vi "FL_Adjust_raw_magnets_coords.vi"(4 "Offset H.":sgl, 5 "Offset V.":sgl, 6 "Alternative magnets orientation":bool, 7 "DEC cluster in":T1) -> (1 "DEC cluster out":T1)   [LabVIEW 2018]
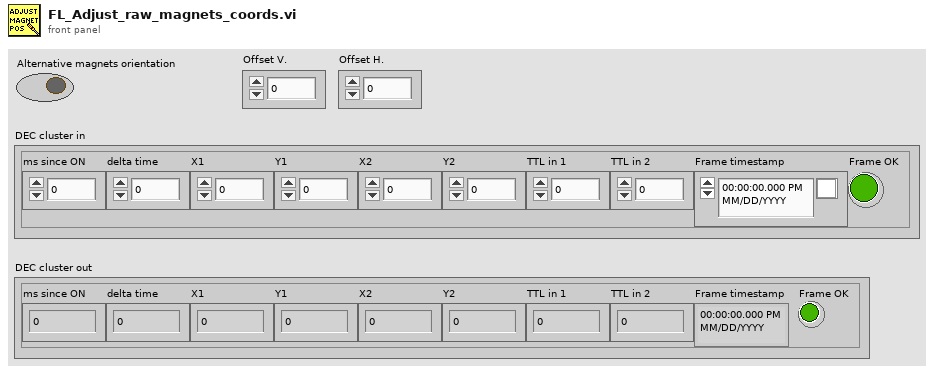
[diagram p1: front panel]
types:
  T1 = cluster{"ms since ON":u32, "delta time":u32, "X1":sgl, "Y1":sgl, "X2":sgl, "Y2":sgl, "TTL in 1":i16, "TTL in 2":i16, "Frame timestamp":timestamp, "Frame OK":bool}
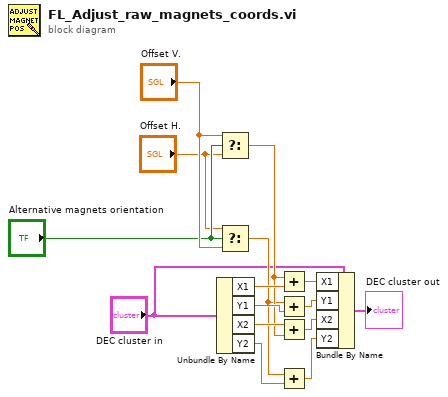
[diagram p0: block diagram]
diagram:
  n1 = Unbundle By Name("DEC cluster in") -> ("X1"=w13:sgl, "Y1"=w15:sgl, "X2"=w12:sgl, "Y2"=w14:sgl)
  n2 = Select(t="Offset V.", s="Alternative magnets orientation", f="Offset H.") -> (s? t:f=w10:sgl)
  n3 = Select(t="Offset H.", s="Alternative magnets orientation", f="Offset V.") -> (s? t:f=w9:sgl)
  n4 = Add(x=w10, y=w13) -> (x+y=w5:sgl)
  n5 = Add(x=w9, y=w15) -> (x+y=w4:sgl)
  n6 = Add(x=w12, y=w10) -> (x+y=w3:sgl)
  n7 = Add(x=w9, y=w14) -> (x+y=w2:sgl)
  n8 = Bundle By Name(cluster="DEC cluster in", "X1"=w5, "Y1"=w4, "X2"=w3, "Y2"=w2) -> (→"DEC cluster out":T1)
